vi "DCMotor.vi"(8 "dt":dbl, 9 "I":dbl, 10 "Omega":dbl, 11 "V":dbl) -> (1 "Torque Out":dbl, 2 "I Out":dbl, 3 "Omega Out":dbl)   [LabVIEW 2016]
uses:
  <vilib>/ptbypt/NI_PtbyPt.lvlib
panel:
  in  "Ng":dbl=8.0
  in  "Cs":dbl=0.03
  in  "Cv":dbl=4e-05
  in  "J":dbl=4e-05
  in  "L":dbl=0.8
  in  "R":dbl=7.0
  in  "K":dbl=0.063
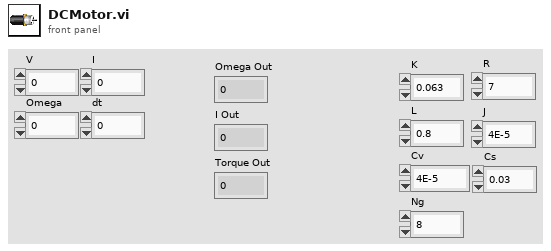
[diagram p1: front panel]
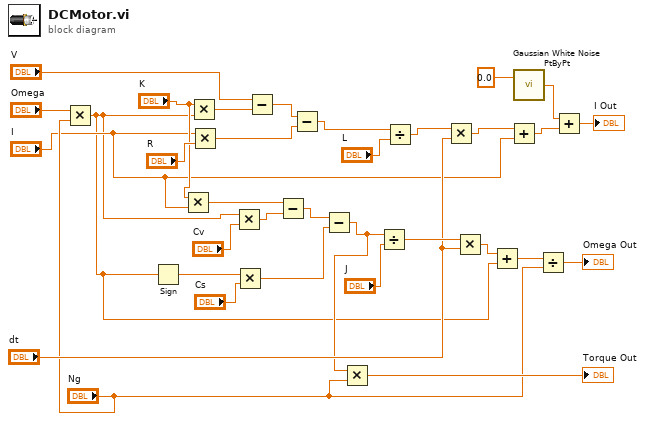
[diagram p0: block diagram]
diagram:
  n1 = Multiply(x="Omega", y="Ng") -> (x*y=w1:dbl)
  n2 = Sign(1:w1) -> (0:w21:dbl)
  n3 = Multiply(x="K", y="I") -> (x*y=w23:dbl)
  n4 = Multiply(x="K", y=w1) -> (x*y=w32:dbl)
  n5 = Multiply(x="I", y="R") -> (x*y=w30:dbl)
  n6 = Multiply(x=w1, y="Cv") -> (x*y=w22:dbl)
  n7 = Multiply(x=w21, y="Cs") -> (x*y=w18:dbl)
  n8 = Subtract(x="V", y=w32) -> (x-y=w31:dbl)
  n9 = Subtract(x=w23, y=w22) -> (x-y=w19:dbl)
  n10 = Subtract(x=w31, y=w30) -> (x-y=w28:dbl)
  n11 = Subtract(x=w19, y=w18) -> (x-y=w13:dbl)
  n12 = Multiply(x=w13, y="Ng") -> (x*y=→"Torque Out":dbl)
  n13 = Divide(x=w13, y="J") -> (x/y=w16:dbl)
  n14 = Divide(x=w28, y="L") -> (x/y=w27:dbl)
  n15 = Multiply(x=w27, y="dt") -> (x*y=w26:dbl)
  n16 = Multiply(x=w16, y="dt") -> (x*y=w14:dbl)
  n17 = Add(x=w14, y=w1) -> (x+y=w10:dbl)
  n18 = Add(x=w26, y="I") -> (x+y=w7:dbl)
  n19 = call <vilib>:"Gaussian White Noise PtByPt.vi"("standard deviation"=0.0 ("amplitude")) -> ("Gaussian white noise"=w5:dbl)  [unwired: 2 in]
  n20 = Divide(x=w10, y="Ng") -> (x/y=→"Omega Out":dbl)
  n21 = Add(x=w5, y=w7) -> (x+y=→"I Out":dbl)
